vi "Launcher Template (Top Level VI).vi"() -> ()   [LabVIEW 2019, in "Architecture.lvlib"]
uses:
  Architecture.lvlib
  Typedefs/FGV Ref. Modules Function.ctl
  Typedefs/Enum_Module_Name.ctl
  Typedefs/Module References.ctl
  Typedefs/Message.ctl
  Modules/Module Template/Module Template.lvlib
panel:
  out "error out":errorcluster
  in  "Loading Bar":u8(slide) caption="Loading Database..." max=100 step=1 scale=0.0..100.0
  # "APPLICATION LAUNCHER"
  # "Juan Pérez Rodríguez"
  # "www.CtrlVIStudios.com"
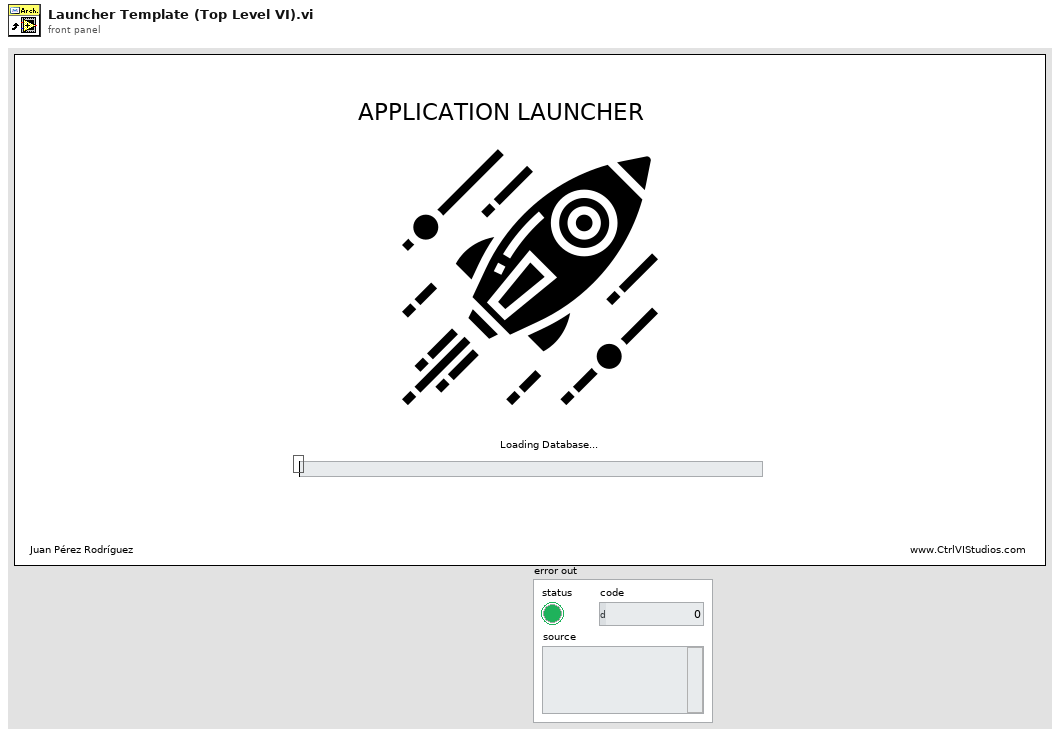
[diagram p1: front panel]
types:
  T1 = typedef "Architecture.lvlib/Enum_Module_Name.ctl" = enum16{"Configuration", "Error_Handler", "Log", "Database", "Controller", "User Console", "Display Console", "Sensor Interface"}
  T2 = cluster{"ModuleName":T1, "ShowFP":bool, "StatesTracking Enabled":bool}[]
  T3 = typedef "Architecture.lvlib/FGV Ref. Modules Function.ctl" = enum16{"Init ", "Add Module", "Get Module", "Get All", "Add Asynchronous Run Ref", "Dispose"}
  T4 = typedef "Architecture.lvlib/Module References.ctl" = cluster{"ModuleName":T1, "Queue":refnum<queue>, "user event":refnum<user-event>, "VI Refnum":refnum<vi>, "ShowFP":bool, "StatesTracking Enabled":bool}
  T5 = enum32{"invalid app kind", "Development System", "Run Time System", "Student Edition", "Embedded LabVIEW", "Evaluation", "Custom"}
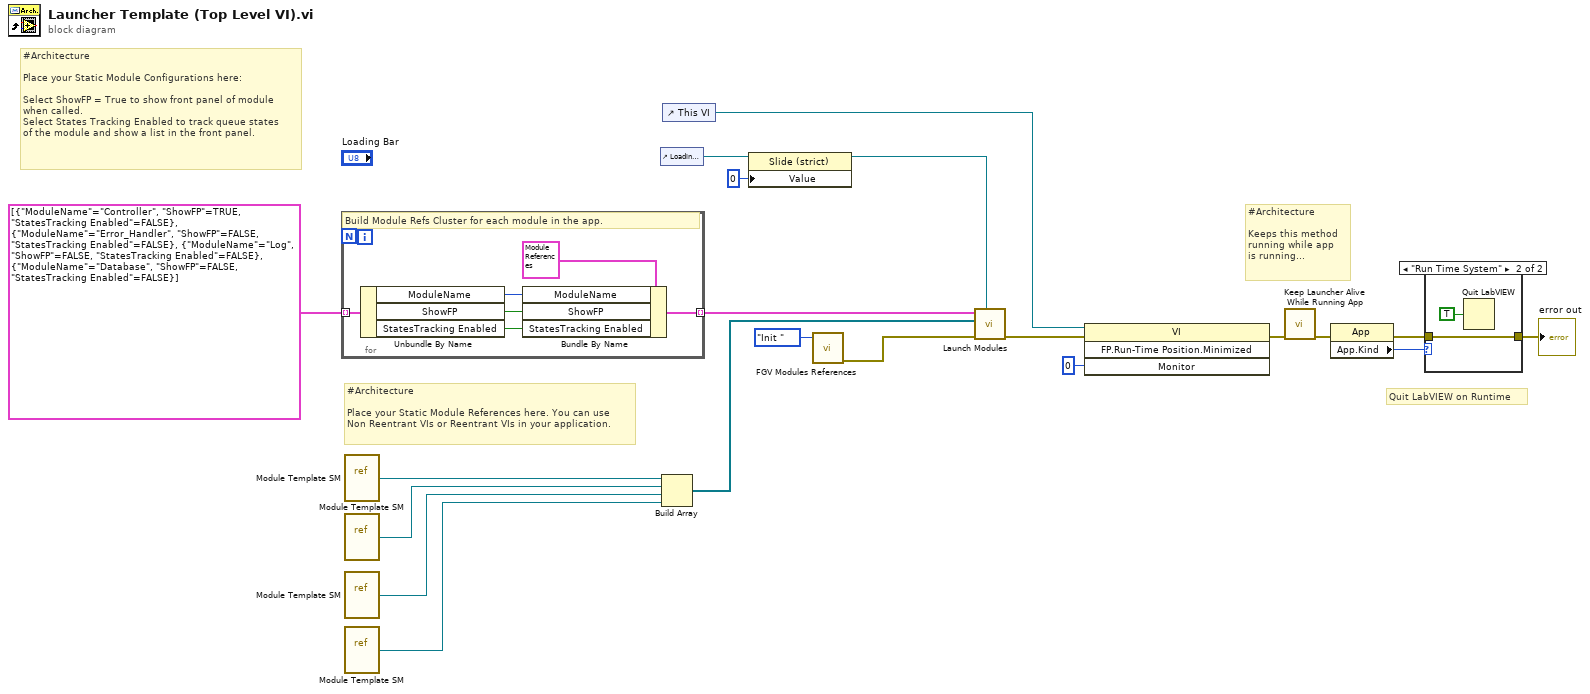
[diagram p0: block diagram]
diagram:
  # "#Architecture\n\nKeeps this method \nrunning while app \nis running..."
  # "Quit LabVIEW on Runtime"
  # "#Architecture\n\nPlace your Static Module References here. You can use\nNon Reentrant VIs or Reentrant VIs in your application."
  # "#Architecture\n\nPlace your Static Module Configurations here:\n\nSelect ShowFP = True to show front panel of module\nwhen called. \nSelect States Tracking Enabled to track queue states\nof the module and show a list in the front panel."
  n1 = for {
    tunnel: T2 [{"ModuleName"=enum."Controller", "ShowFP"=TRUE, "StatesTracking Enabled"=FALSE}, {"ModuleName"=enum."Error_Handler", "ShowFP"=FALSE, "StatesTracking Enabled"=FALSE}, {"ModuleName"=enum."Log", "ShowFP"=FALSE, "StatesTracking Enabled"=FALSE}, {"ModuleName"=enum."Database", "ShowFP"=FALSE, "StatesTracking Enabled"=FALSE}] -> [w25] mode=indexing
    tunnel: [w21] -> w19 mode=indexing
    # "Build Module Refs Cluster for each module in the app."
    n2 = Unbundle By Name(w25) -> ("ModuleName"=w24:T1, "ShowFP"=w23:bool, "StatesTracking Enabled"=w22:bool)
    n3 = Bundle By Name(cluster=T4 {"ModuleName"=enum."Controller", "Queue"=refnum, "user event"=refnum, "VI Refnum"=refnum, "ShowFP"=FALSE, "StatesTracking Enabled"=FALSE} ("Module_Refs"), "ModuleName"=w24, "ShowFP"=w23, "StatesTracking Enabled"=w22) -> (w21:T4)
  }
  n4 = vi-ref "Module Template SM.vi"() -> (w7:refnum<vi>)
  n5 = vi-ref "Module Template SM.vi"() -> (w6:refnum<vi>)
  n6 = vi-ref "Module Template SM.vi"() -> (w5:refnum<vi>)
  n7 = vi-ref "Module Template SM.vi"() -> (w4:refnum<vi>)
  n8 = control-ref of="Loading Bar"() -> (w18:refnum<vi>)
  n9 = Build Array(w7, w6, w5, w4) -> (w12:refnum<vi>[])
  n10 = control-ref of="This VI"() -> (w11:refnum<vi>)
  n11 = property class="Slide (strict)"(reference=w18, "Value"=u8 0) -> (reference out=w15:refnum<vi>)  [unwired: 1 in, 1 out]
  n12 = call "FGV Modules References.vi"("FGV Ref. Function In"=FGV_Ref._Modules_Function."Init ") -> ("error out"=w16:errorcluster)  [unwired: 8 in, 2 out]
  n13 = call "Launch Modules.vi"("Loading Bar Ref In"=w15, "error in (no error)"=w16, "App Modules Refs"=w12, "Modules Info In"=w19) -> ("error out"=w13:errorcluster)  [unwired: 7 in]
  n14 = invoke class="VI" method="FP.Run-Time Position.Minimized"(reference=w11, error in=w13, "Monitor"=i16 0) -> (error out=w10:errorcluster)  [unwired: 1 in, 3 out]
  n15 = call "Keep Launcher Alive While Running App.vi"("error in (no error)"=w10) -> ("error out"=w9:errorcluster)  [unwired: 10 in]
  n16 = property class="App"(error in=w9) -> (error out=w3:errorcluster, "App.Kind"=w1:T5)  [unwired: 1 in, 1 out]
  n17 = case shown="\"Run Time System\"" w1 {
    tunnel: w3 -> [w27 w29]
    tunnel: [w27 w29] -> w2
    frame Default {
    }
    frame "Run Time System" {
      n18 = Quit LabVIEW(quit? (T)=TRUE) -> ()
    }
  }
  "error out" <- w2
